vi "AOselector.vi"(8 "I/O element":enum16{""}(ring), 11 "value":i16) -> ()   [LabVIEW 2024]
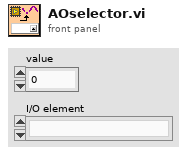
[diagram p1: front panel]
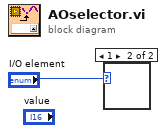
[diagram p0: block diagram]
diagram:
  n1 = case shown="\"1\"" "I/O element" {
    frame "", Default {
    }
    frame 1 {
    }
  }
